vi "startSerial.vi"(8 "error in (no error)":errorcluster, 11 "EncoderReader in":refnum<class "EncoderReader.lvclass">) -> (0 "error out":errorcluster, 3 "EncoderReader out":refnum<class "EncoderReader.lvclass">)   [LabVIEW 2013, in "EncoderReader.lvlib" / "EncoderReader.lvclass"]
uses:
  <userlib>/Common/Devices/EncoderReader/EncoderReader/EncoderReader.lvclass
  <userlib>/Common/Devices/EncoderReader/EncoderReader/EncoderReader.lvclass/EncoderReader.ctl
  <userlib>/Common/SerialProtocols/SerialCommunicator/SerialCommunicator.lvclass
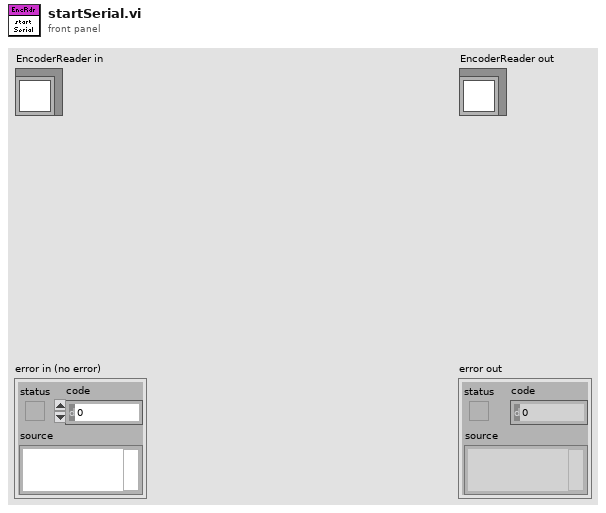
[diagram p1: front panel]
types:
  T1 = typedef "SerialProtocols.lvlib/SerialConfig.ctl" = cluster{"Serial Protocol":T2, "Protocol Parameters":T3, "Serial Message Parameters":T4}
  T2 = typedef "SerialProtocols.lvlib/SerialProtocol.ctl" = enum16{"RS232", "RS485", "SerialSimulator"}
  T3 = typedef "SerialProtocols.lvlib/ProtocolParameters.ctl" = cluster{"VISA resource name":refnum<visa-resource-name>, "Baud Rate":u32, "Data Bits":u16, "Parity":enum16{"None", "Odd", "Even", "Mark", "Space"}, "Flow Control":u16, "Stop Bits":u16, "Timeout (ms)":u32}
  T4 = typedef "SerialProtocols.lvlib/SerialMessageParameters.ctl" = cluster{"Byte Count":u32, "Enable Termination Character":bool, "Termination Char":u8}
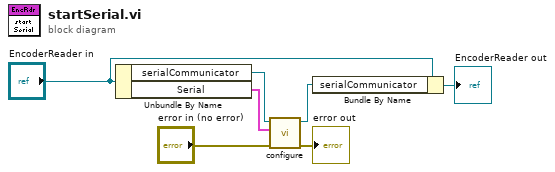
[diagram p0: block diagram]
diagram:
  n1 = Unbundle By Name("EncoderReader in") -> ("serialCommunicator"=w6:refnum<class "SerialCommunicator.lvclass">, "Serial"=w7:T1)
  n2 = call-dynamic "configure.vi"("error in (no error)"="error in (no error)", "SerialConfig"=w7, "SerialCommunicator in"=w6) -> ("error out"=→"error out":errorcluster, "SerialCommunicator out"=w5:refnum<class "SerialCommunicator.lvclass">)  [unwired: 7 in]
  n3 = Bundle By Name(cluster="EncoderReader in", "serialCommunicator"=w5) -> (→"EncoderReader out":refnum<class "EncoderReader.lvclass">)
